vi "Reset.vi"(8 "error in (no error)":errorcluster, 11 "device in":tag) -> (0 "error out":errorcluster)   [LabVIEW 2020, in "niMIO.lvclass"]
uses:
  niMIO.lvclass
panel:
  out "niDIO out":refnum<class "niMIO.lvclass">
  in  "niDIO in":refnum<class "niMIO.lvclass">
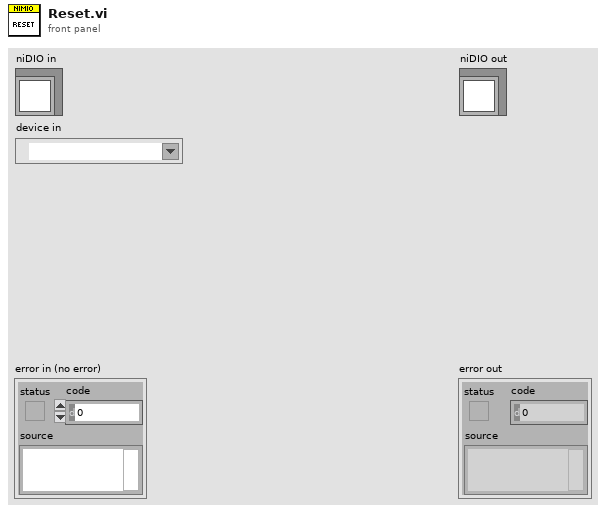
[diagram p1: front panel]
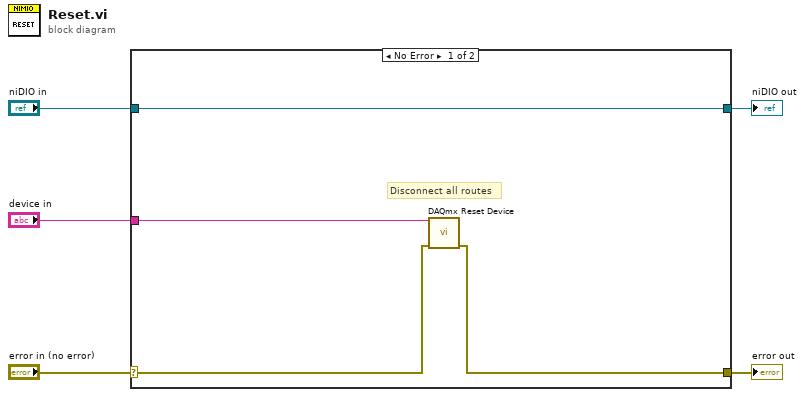
[diagram p0: block diagram]
diagram:
  n1 = case shown="No Error" "error in (no error)" {
    selector: "error in (no error)" -> [w8 w11]
    tunnel: [w7 w11] -> w4
    tunnel: [w9 w10] -> w2
    tunnel: "niDIO in" -> [w9 w10]
    tunnel: "device in" -> [w6 _]
    frame No Error {
      # "Disconnect all routes"
      n2 = call <vilib>:"DAQmx Reset Device.vi"("device in"=w6, "error in"=w8) -> ("error out"=w7:errorcluster)  [unwired: 13 in]
    }
    frame Error {
    }
  }
  "error out" <- w4
  "niDIO out" <- w2
